vi "setResults.vi"(8 "error in (no error)":errorcluster, 10 "results":T1, 11 "ImageAnalyser in":refnum<class "ImageAnalyser.lvclass">) -> (0 "error out":errorcluster, 3 "ImageAnalyser out":refnum<class "ImageAnalyser.lvclass">)   [LabVIEW 2011, in "Tools.lvlib" / "Imaging.lvlib" / "ImageAnalyser.lvclass"]
uses:
  ImageAnalyser.lvclass
  ImageAnalyser.lvclass/ImageAnalyser.ctl
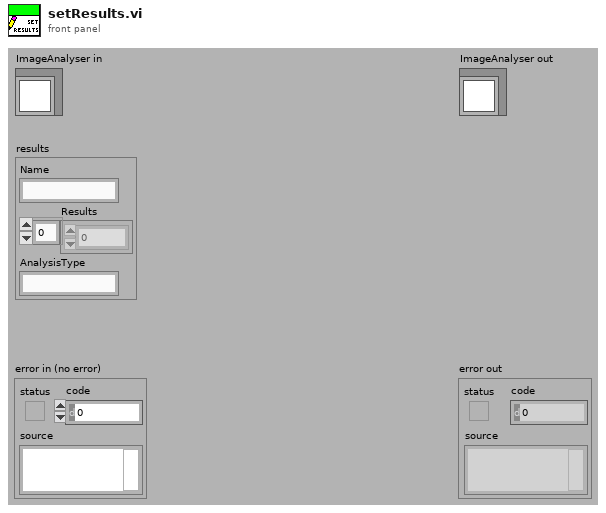
[diagram p1: front panel]
types:
  T1 = cluster{"Name":string, "Results":dbl[], "AnalysisType":string}
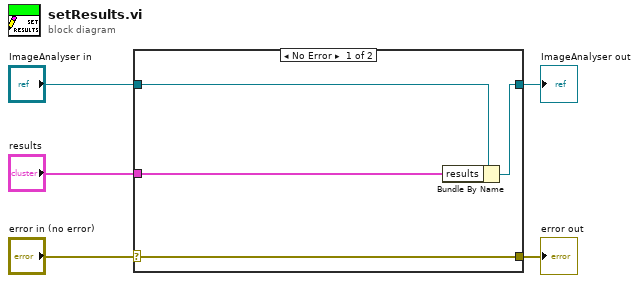
[diagram p0: block diagram]
diagram:
  n1 = case shown="No Error" "error in (no error)" {
    selector: "error in (no error)" -> [w9 w10]
    tunnel: [w9 w10] -> w4
    tunnel: [w7 w11] -> w2
    tunnel: "ImageAnalyser in" -> [w8 w11]
    tunnel: "results" -> [w6 _]
    frame No Error {
      n2 = Bundle By Name(cluster=w8, "results"=w6) -> (w7:refnum<class "ImageAnalyser.lvclass">)
    }
    frame Error {
    }
  }
  "error out" <- w4
  "ImageAnalyser out" <- w2
